vi "RT Driver VI.vi"(6 "Device Clock":string, 9 "Device Inputs FIFO":refnum<k33>, 10 "Device Outputs FIFO":refnum<k33>, 11 "Device Reference":T1 format="%.0x") -> ()   [LabVIEW 2020, in "NI PXIe-4340 Engine.lvlib"]
uses:
  NI PXIe-4340 Engine.lvlib
  <vilib>/NI VeriStand/Custom Device API/Custom Device Item Ref.ctl
  <vilib>/NI VeriStand/Custom Device API/Custom Device Channel Type.ctl
  <vilib>/NI VeriStand/Custom Device API/Message Response (String).ctl
  <vilib>/NI VeriStand/Custom Device API/Message Response (Byte Array).ctl
  <vilib>/DAQmx/read.llb/DAQmx Read (Analog 1D DBL NChan 1Samp).vi
  Shared/Constants.vi
  <vilib>/DAQmx/miscellaneous.llb/DAQmx Fill In Error Info.vi
  <vilib>/NI VeriStand/Custom Device API/Custom Device API.lvlib
  <vilib>/NI VeriStand/Custom Device Tools/Custom Device Utility Library/Custom Device Utility Library.lvlib
  Shared/NI PXIe-4340 Shared.lvlib
panel:
  in  "Initialization Status Notifier":refnum<notifier>
  in  "Status Notifier":refnum<notifier>
  # "Custom Device Template\nv1.0"
  # "Use this template as a starting point for creating a custom device code module. The input controls shown here are specially named controls that the system will use to provide the device loop with data. The controls are not required for the device loop to run. For instance, if the device doesn't produce any output data, then you don't need the Device Outputs FIFO control. If you do use these controls, however, they need to have these exact names to be functional."
  # "The optional status notifier element is used to notify the RT engine of the last state of the custom device, and to indicate the device has completed execution. If this control is not used, a default No Error value is returned to the system when the device finishes execution.\n\nNote: This error state is not checked until the system shuts down. Use an output status channel to send more immediate status values to the system."
  # "This optional input can be used to send the VeriStand Engine the final status of the custom device initalization process. If this control exists on the custom device front panel, the VeriStand Engine will wait for a status update before starting up. If the custom device reports an error, that will abort the execution of the current configuration in the VeriStand Engine.\n\nThis control can be deleted if the custom device does not need to send the initialization status update."
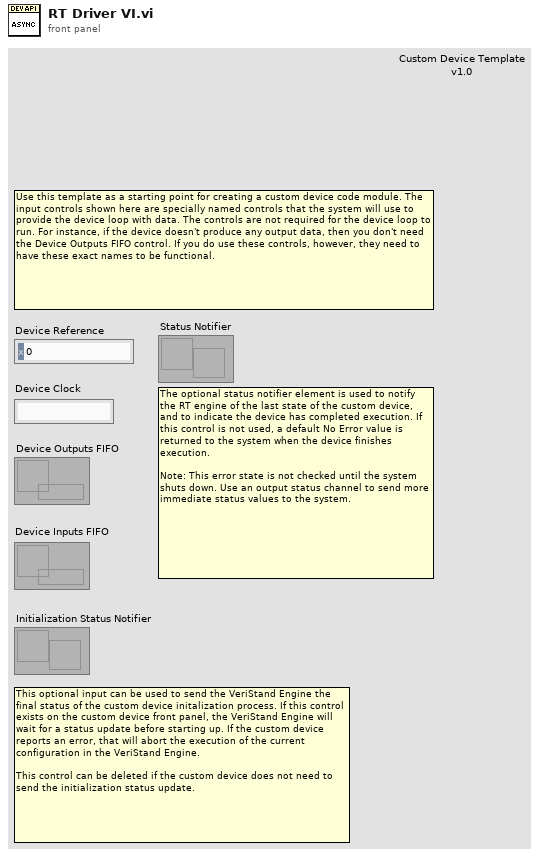
[diagram p1: front panel]
types:
  T1 = typedef "Custom Device API.lvlib/Custom Device Item Ref.ctl" = u64
  T2 = typedef "Custom Device API.lvlib/Custom Device Channel Type.ctl" = enum16{"Input", "Output"}
  T3 = typedef "Custom Device API.lvlib/Custom Device Engine Event Ref.ctl" = refnum<event-registration>
  T4 = typedef "Custom Device API.lvlib/Message Response (String).ctl" = cluster{"Response":string, "Error":errorcluster}
  T5 = typedef "Custom Device API.lvlib/Message Response (Byte Array).ctl" = cluster{"Response":u8[], "Error":errorcluster}
  T6 = typedef "NI PXIe-4340 Shared.lvlib/Device Configuration.ctl" = cluster{"Device Name":string, "Sample Rate (Hz)":dbl, "Enabled Channels":bool[]}
  T7 = typedef "NI PXIe-4340 Shared.lvlib/Channel Configuration.ctl" = cluster{"Channel#":i32, "Measurement Type":i32, "Position_LVDT_Properties":T8, "Position_RVDT_Properties":T9}
  T8 = typedef "NI PXIe-4340 Shared.lvlib/Position_LVDT_Properties.ctl" = cluster{"Minimum Value":dbl, "Maximum Value":dbl, "Excitation Source":i32, "Excitation Wire Mode":i32, "Excitation Frequency":dbl, "Excitation Value":dbl, "Units":i32, "Sensitivity":dbl, "Sensitivity Units":i32, "Excitation Sense":i32}
  T9 = typedef "NI PXIe-4340 Shared.lvlib/Position_RVDT_Properties.ctl" = cluster{"Minimum Value":dbl, "Maximum Value":dbl, "Excitation Source":i32, "Excitation Wire Mode":i32, "Excitation Frequency":dbl, "Excitation Value":dbl, "Units":i32, "Sensitivity":dbl, "Sensitivity Units":i32, "Excitation Sense":i32}
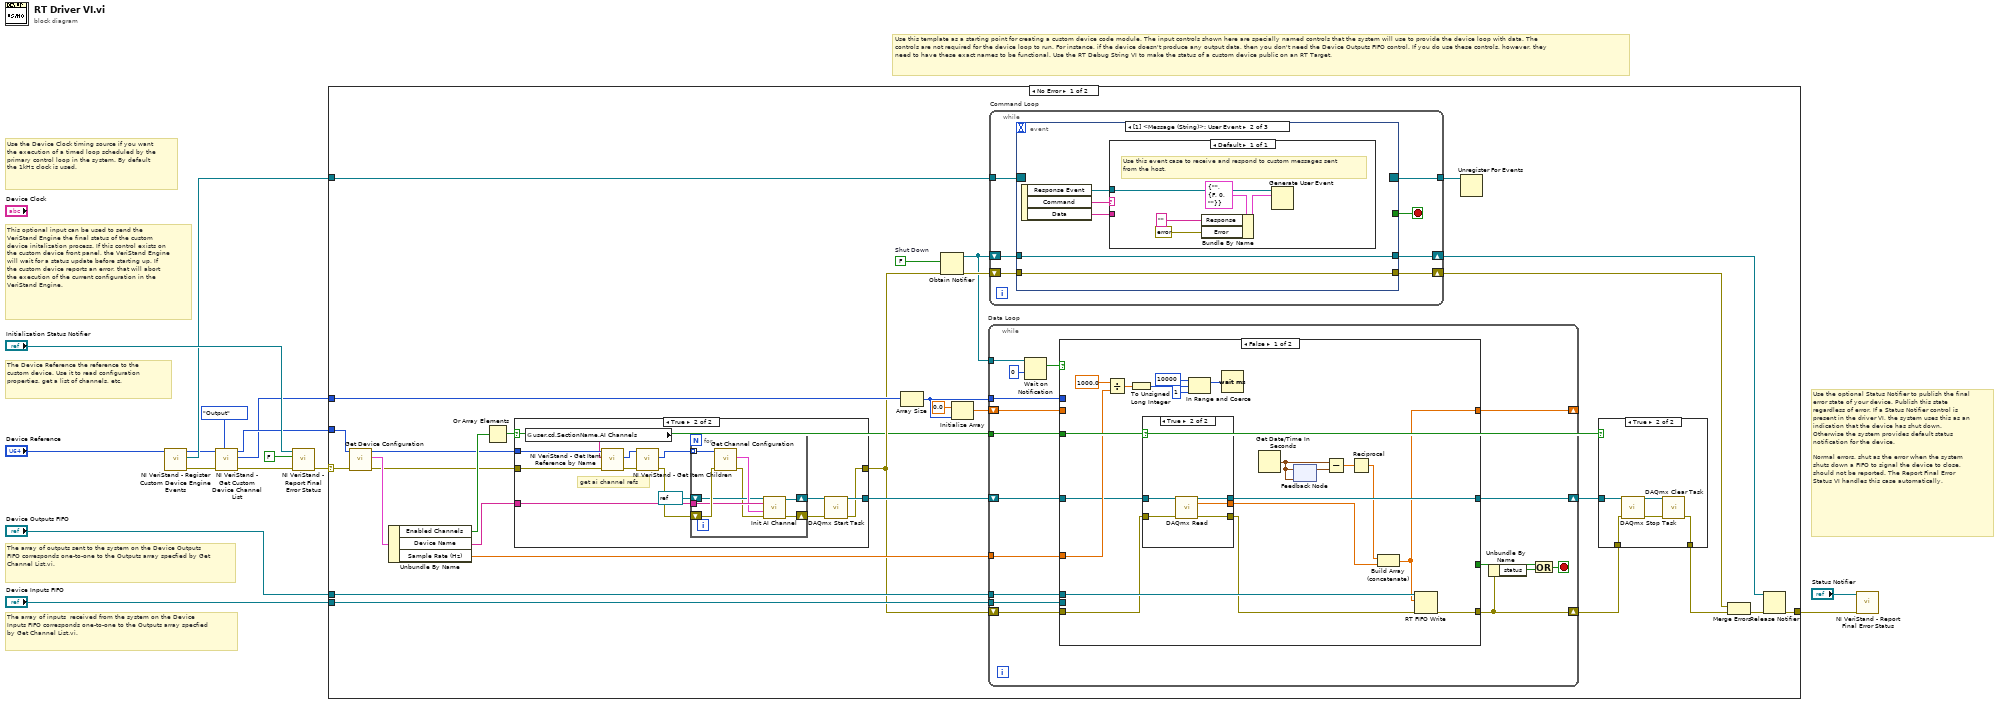
[diagram p0: block diagram]
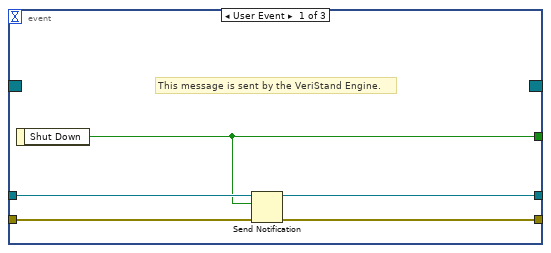
[diagram p4: hidden frame]
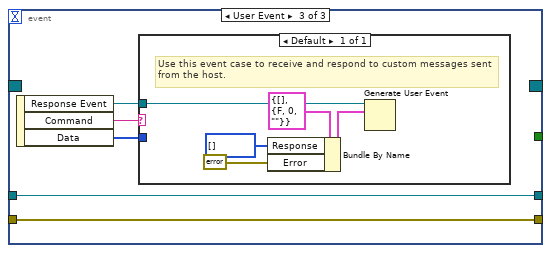
[diagram p5: hidden frame]
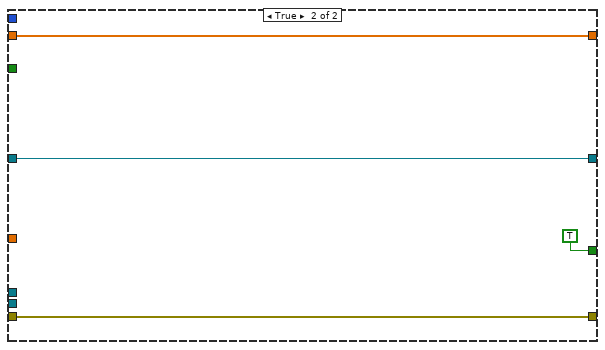
[diagram p7: hidden frame]
diagram:
  # "This optional input can be used to send the VeriStand Engine the final status of the custom device initalization process. If this control exists on the custom device front panel, the VeriStand Engine will wait for a status update before starting up. If the custom device reports an error, that will abort the execution of the current configuration in the VeriStand Engine."
  # "The array of inputs  received from the system on the Device Inputs FIFO corresponds one-to-one to the Outputs array specfied by Get Channel List.vi."
  # "Use the optional Status Notifier to publish the final error state of your device. Publish this state regardless of error. If a Status Notifier control is present in the driver VI, the system uses this as an indication that the device has shut down. Otherwise the system provides default status notification for the device.\n\nNormal errors, shut as the error when the system shuts down a FIFO to signal the device to close, should not be reported. The Report Final Error Status VI handles this case automatically."
  # "The array of outputs sent to the system on the Device Outputs FIFO corresponds one-to-one to the Outputs array specfied by Get Channel List.vi."
  # "The Device Reference the reference to the custom device. Use it to read configuration properties, get a list of channels, etc."
  # "Use the Device Clock timing source if you want the execution of a timed loop scheduled by the primary control loop in the system. By default the 1kHz clock is used."
  # "Use this template as a starting point for creating a custom device code module. The input controls shown here are specially named controls that the system will use to provide the device loop with data. The controls are not required for the device loop to run. For instance, if the device doesn't produce any output data, then you don't need the Device Outputs FIFO control. If you do use these controls, however, they need to have these exact names to be functional. Use the RT Debug String VI to make the status of a custom device public on an RT Target."
  n1 = call <vilib>:"NI VeriStand - Register Custom Device Engine Events.vi"("Device Ref in"="Device Reference") -> ("error out"=w15:errorcluster, "Custom Device Engine Event Ref"=w7:T3, "Device Ref out"=w4:T1)  [unwired: 8 in]
  n2 = call <vilib>:"NI VeriStand - Get Custom Device Channel List.vi"("Channel Type"=Custom_Device_Channel_Type."Output", "error in (no error)"=w15, "Device Ref in"=w4) -> ("error out"=w9:errorcluster, "Specified Channel Ref List"=w1:T1[], "Device Ref out"=w10:T1)  [unwired: 6 out]
  n3 = call <vilib>:"NI VeriStand - Report Final Error Status.vi"("error in (no error)"=w9, "Filter FIFO & Shutdown Errors (T)"=FALSE ("Filter FIFO Errors (T)"), "Status Notifier"="Initialization Status Notifier") -> ("error out"=w3:errorcluster)  [unwired: 8 out]
  n4 = case shown="No Error" w3 {
    selector: w3 -> [w21 w153]
    tunnel: "Device Outputs FIFO" -> [w43 _]
    tunnel: "Device Inputs FIFO" -> [w42 _]
    tunnel: w1 -> [w27 _]
    tunnel: w7 -> [w39 _]
    tunnel: [w37 w153] -> w6
    tunnel: w10 -> [w28 _]
    frame No Error {
      w38 = FALSE  # Shut Down
      n5 = call "Get Device Configuration.vi"("error in (no error)"=w21, "Device Item Ref in"=w28) -> ("error out"=w17:errorcluster, "Device Configuration"=w30:T6, "Device Item Ref out"=w16:T1)  [unwired: 7 in]
      n6 = Unbundle By Name(w30) -> ("Enabled Channels"=w19:bool[], "Device Name"=w29:string, "Sample Rate (Hz)"=w26:dbl)
      n7 = Or Array Elements(Boolean array=w19) -> (logical OR=w18:bool)
      n8 = case shown="True" w18 {
        tunnel: w29 -> [_ w58]
        tunnel: [_ w55] -> w25
        tunnel: [w45 w53] -> w20
        tunnel: w17 -> [w45 w50]
        tunnel: w16 -> [_ w49]
        frame False {
        }
        frame True {
          # "get ai channel refs"
          n9 = global read "Constants.vi" "user.cd.SectionName.AI Channels"() -> (w46:string)
          n10 = call <vilib>:"NI VeriStand - Get Item Reference by Name.vi"("error in (no error)"=w50, "Item Name"=w46, "Parent Ref in"=w49) -> ("error out"=w52:errorcluster, "Item Ref"=w51:T1)  [unwired: 5 in, 2 out]
          n11 = call <vilib>:"NI VeriStand - Get Item Children.vi"("error in (no error)"=w52, "Item Ref in"=w51) -> ("error out"=w48:errorcluster, "Child Refs"=w47:T1[])  [unwired: 6 in, 2 out]
          n12 = for {
            tunnel: w58 -> [w65]
            tunnel: w47 -> [w64] mode=indexing
            shift-right: [w62] -> w56
            shift-left: refnum<k21> refnum ("task out") -> [w61]
            shift-right: [w59] -> w54
            shift-left: w48 -> [w66]
            n13 = call "Get Channel Configuration.vi"("error in (no error)"=w66, "Channel Item Ref in"=w64) -> ("error out"=w60:errorcluster, "Channel Configuration"=w63:T7)  [unwired: 7 in, 1 out]
            n14 = call "Init AI Channel.vi"("error in"=w60, "Channel Configuration"=w63, "Device Name"=w65, "task in"=w61) -> ("error out"=w59:errorcluster, "task out"=w62:refnum<k21>)  [unwired: 6 in]
          }
          n15 = call <vilib>:"DAQmx Start Task.vi"("task/channels in"=w56, "error in"=w54) -> ("task out"=w55:refnum<k21>, "error out"=w53:errorcluster)  [unwired: 12 in]
        }
      }
      n16 = Array Size(array=w27) -> (size(s)=w40:i32)
      n17 = Obtain Notifier(notification data type=w38, error in (no error)=w20) -> (notifier out=w35:refnum<notifier>, error out=w44:errorcluster)  [unwired: 2 in, 1 out]
      n18 = Initialize Array(0.0 ("element"), w40) -> (w41:dbl[])
      n19 = while "Data Loop" {
        shift-right: [w114] -> w23
        shift-left: w20 -> [w121]
        shift-right: [w119] -> _
        shift-left: w41 -> [w120]
        tunnel: w40 -> [w116]
        tunnel: w43 -> [w118]
        tunnel: w42 -> [w117]
        tunnel: w35 -> [w113]
        tunnel: w26 -> [w108]
        shift-right: [w106] -> w24
        shift-left: w25 -> [w107]
        tunnel: w18 -> [w105]
        stop <- w109 stop-if-true
        n20 = Wait on Notification(notifier=w113, timeout in ms (-1)=0) -> (notification=w112:bool)  [unwired: 2 in, 3 out]
        n21 = case shown="False" w112 {
          tunnel: w121 -> [w127 w152]
          tunnel: w120 -> [_ w151]
          tunnel: [w122 w151] -> w119
          tunnel: w118 -> [w141 _]
          tunnel: w117 -> [_ _]
          tunnel: w116 -> [_ _]
          tunnel: [w140 w152] -> w114
          tunnel: [_ TRUE] -> w110
          tunnel: w108 -> [w137 _]
          tunnel: w107 -> [w130 w149]
          tunnel: [w128 w149] -> w106
          tunnel: w105 -> [w129 _]
          frame False {
            n22 = Divide(x=1000.0, y=w137) -> (x/y=w136:dbl)
            n23 = To Unsigned Long Integer(number=w136) -> (unsigned 32bit integer=w134:u32)
            n24 = case shown="True" w129 {
              tunnel: w130 -> [w143 w148]
              tunnel: [w143 w147] -> w128
              tunnel: w127 -> [w142 w146]
              tunnel: [w142 w145] -> w126
              tunnel: [_ w144] -> w125
              frame False {
              }
              frame True {
                n25 = call-poly <vilib>:"DAQmx Read.vi"("task/channels in"=w148, "error in"=w146) -> ("task out"=w147:refnum<k21>, "data"=w144:dbl[], "error out"=w145:errorcluster)  [unwired: 11 in]
              }
            }
            n26 = In Range and Coerce(upper limit=u32 10000, x=w134, lower limit=u32 1) -> (coerced(x)=w131:u32)  [unwired: 1 out]
            n27 = Wait (ms)(milliseconds to wait=w131) -> ()  [unwired: 1 out]
            n28 = Get Date/Time In Seconds() -> (seconds since 1Jan1904=w138:timestamp)
            n29 = feedback #1(w138) -> (w139:timestamp)
            n30 = feedback-in #1(w138) -> ()
            n31 = Subtract(x=w138, y=w139) -> (x-y=w124:dbl)
            n32 = Reciprocal(x=w124) -> (1/x=w123:dbl)
            n33 = Build Array (concatenate)(w123, w125) -> (w122:dbl[])
            n34 = RT FIFO Write(0:w141, 1:w122, 3:w126) -> (11:w140:errorcluster)  [unwired: 1 in, 4 out]
          }
          frame True {
          }
        }
        n35 = Unbundle By Name(w114) -> ("status"=w111:bool)
        n36 = Compound Arithmetic op=OR(w110, w111) -> (w109:bool)
      }
      n37 = while "Command Loop" {
        tunnel: w39 -> [w79]
        tunnel: [w78] -> w36
        shift-right: [w75] -> w34
        shift-left: w35 -> [w76]
        shift-right: [w73] -> w32
        shift-left: w44 -> [w74]
        stop <- w77 stop-if-true
        n38 = event shown="[1] <Message (String)>: User Event" {
          selector: w79 -> [_ _ _]
          dyn-events: [_ _ _] -> w78
          timeout: _ -> [_ _ _]
          tunnel: [w82 _ _] -> w77
          tunnel: w76 -> [w83 w87 w97]
          tunnel: [w84 w87 w97] -> w75
          tunnel: w74 -> [w81 w85 w95]
          tunnel: [w80 w85 w95] -> w73
          event User Event {
            # "This message is sent by the VeriStand Engine."
            n39 = event-data() -> ("Shut Down"=w82:bool)  [unwired: 1 in]
            n40 = Send Notification(notification=w82, notifier=w83, error in (no error)=w81) -> (notifier out=w84:refnum<notifier>, error out=w80:errorcluster)
          }
          event User Event {
            n41 = event-data() -> ("Response Event"=w86:refnum<user-event>, "Command"=w89:string, "Data"=w88:string)  [unwired: 1 in]
            n42 = case shown="Default" w89 {
              tunnel: w88 -> [_]
              tunnel: w86 -> [w94]
              frame Default {
                # "Use this event case to receive and respond to custom messages sent from the host."
                n43 = Bundle By Name(cluster=T4 {"Response"="", "Error"={"status"=FALSE, "code"=0, "source"=""}} ("event data"), "Response"="", "Error"=errorcluster {"status"=FALSE, "code"=0, "source"=""}) -> (w92:T4)
                n44 = Generate User Event(user event=w94, event data cluster=w92) -> ()  [unwired: 2 in, 2 out]
              }
            }
          }
          event User Event {
            n45 = event-data() -> ("Response Event"=w96:refnum<user-event>, "Command"=w99:string, "Data"=w98:u8[])  [unwired: 1 in]
            n46 = case shown="Default" w99 {
              tunnel: w98 -> [_]
              tunnel: w96 -> [w104]
              frame Default {
                # "Use this event case to receive and respond to custom messages sent from the host."
                n47 = Bundle By Name(cluster=T5 {"Response"=[], "Error"={"status"=FALSE, "code"=0, "source"=""}} ("event data"), "Response"=u8[] [], "Error"=errorcluster {"status"=FALSE, "code"=0, "source"=""}) -> (w101:T5)
                n48 = Generate User Event(user event=w104, event data cluster=w101) -> ()  [unwired: 2 in, 2 out]
              }
            }
          }
        }
      }
      n49 = Unregister For Events(event registration refnum=w36) -> ()  [unwired: 1 in, 1 out]
      n50 = case shown="True" w18 {
        tunnel: w24 -> [_ w70]
        tunnel: w23 -> [w67 w69]
        tunnel: [w67 w68] -> w22
        frame False {
        }
        frame True {
          n51 = call <vilib>:"DAQmx Stop Task.vi"("task/channels in"=w70, "error in"=w69) -> ("task out"=w72:refnum<k21>, "error out"=w71:errorcluster)  [unwired: 12 in]
          n52 = call <vilib>:"DAQmx Clear Task.vi"("task in"=w72, "error in"=w71) -> ("error out"=w68:errorcluster)  [unwired: 13 in]
        }
      }
      n53 = Merge Errors(w32, w22) -> (w33:errorcluster)
      n54 = Release Notifier(notifier=w34, error in (no error)=w33) -> (error out=w37:errorcluster)  [unwired: 1 in, 2 out]
    }
    frame Error {
    }
  }
  n55 = call <vilib>:"NI VeriStand - Report Final Error Status.vi"("error in (no error)"=w6, "Status Notifier"="Status Notifier") -> ()  [unwired: 1 in, 9 out]
